vi "TOP BOTTOM Timestamp.vi"(4 "Format":enum16{"at TOP", "at BOTTOM", "none"}(ring), 5 "Plot Bounds":T2, 6 "Timestamp":dbl, 7 "pixel center":cluster{"horizontal":i16, "vertical":i16}, 8 "time format (%H:%M:%S)":string="%I:%M:%S %p", 9 "GraphBGK":u32(colorbox), 10 "font":T1, 11 "new picture in":picture) -> (3 "new picture out":picture)   [LabVIEW 2019]
uses:
  <vilib>/Utility/miscctls.llb/LVRectTypeDef.ctl
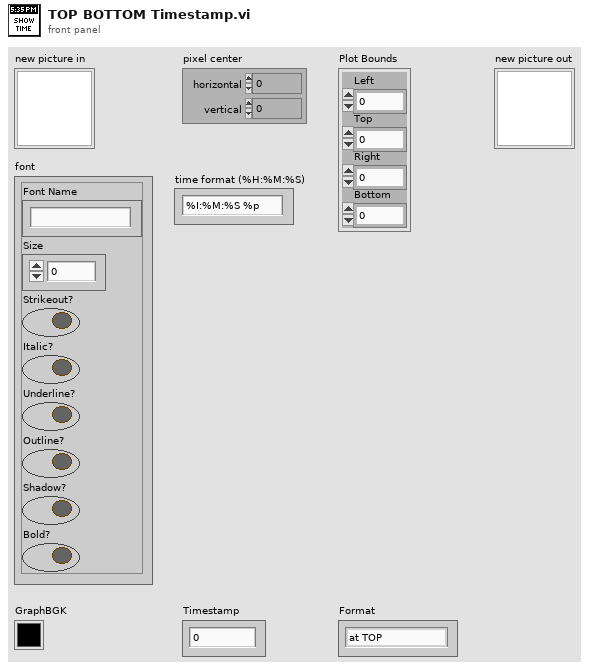
[diagram p1: front panel]
types:
  T1 = cluster{"Font Name":string, "Size":i16, "Strikeout?":bool, "Italic?":bool, "Underline?":bool, "Outline?":bool, "Shadow?":bool, "Bold?":bool}
  T2 = typedef "LVRectTypeDef.ctl" = cluster{"Left":i16, "Top":i16, "Right":i16, "Bottom":i16}
  T3 = enum16{"User-specified Font", "Application Font", "System Font", "Dialog Font"}
  T4 = cluster{"horizontal":enum16{"left", "center", "right"}, "vertical":enum16{"top", "center", "bottom"}}
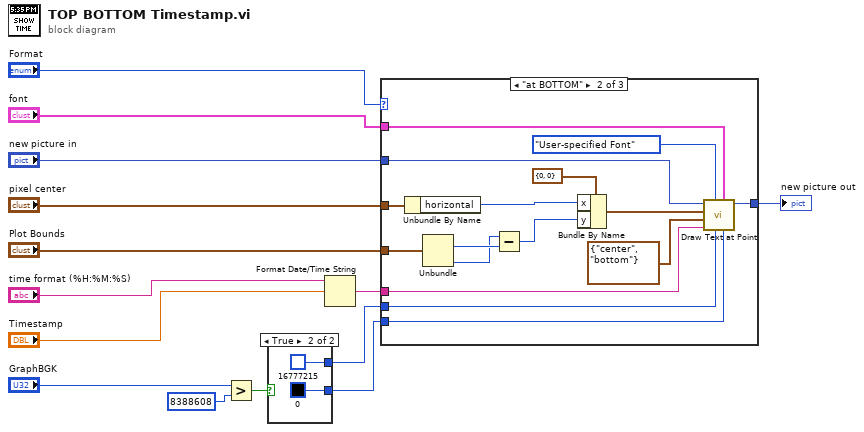
[diagram p0: block diagram]
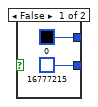
[diagram p2: hidden frame]
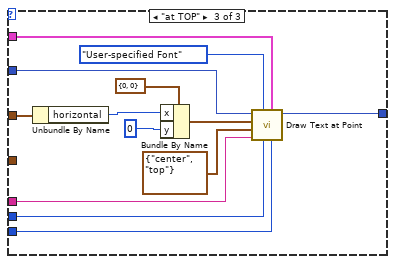
[diagram p4: hidden frame]
diagram:
  n1 = Greater?(x="GraphBGK", y=u32 8388608) -> (0:w9:bool)
  n2 = case shown="True" w9 {
    tunnel: [u32 0 u32 16777215] -> w6
    tunnel: [u32 16777215 u32 0] -> w5
    frame False {
    }
    frame True {
    }
  }
  n3 = Format Date/Time String(time format string (%c)="time format (%H:%M:%S)", seconds (now)="Timestamp") -> (date/time string=w1:string)  [unwired: 1 in]
  n4 = case shown="\"at BOTTOM\"" "Format" {
    tunnel: w1 -> [_ w20 w36]
    tunnel: "Plot Bounds" -> [_ w29 _]
    tunnel: "pixel center" -> [_ w28 w48]
    tunnel: [w19 w34 w46] -> w11
    tunnel: "new picture in" -> [w19 w33 w45]
    tunnel: w6 -> [_ w24 w40]
    tunnel: w5 -> [_ w23 w39]
    tunnel: "font" -> [_ w21 w38]
    frame "none" {
    }
    frame "at BOTTOM" {
      n5 = Unbundle By Name(w28) -> ("horizontal"=w31:i16)
      n6 = Unbundle(w29) -> ("Top"=w27:i16, "Bottom"=w26:i16)  [unwired: 2 out]
      n7 = Subtract(x=w26, y=w27) -> (x-y=w25:i16)
      n8 = Bundle By Name(cluster=cluster{"x":i16, "y":i16} {"x"=0, "y"=0} ("origin"), "x"=w31, "y"=w25) -> (w32:cluster{"x":i16, "y":i16})
      n9 = call <vilib>:"Draw Text at Point.vi"("BG color(transparent)"=w23, "[user-specified font]"=w21, "text color(black)"=w24, "desired font(Application)"=T3."User-specified Font", "text"=w20, "alignment(left, top)"=T4 {"horizontal"=enum."center", "vertical"=enum."bottom"}, "origin"=w32, "picture"=w33) -> ("new picture"=w34:picture)  [unwired: 2 in, 1 out]
    }
    frame "at TOP" {
      n10 = Unbundle By Name(w48) -> ("horizontal"=w43:i16)
      n11 = Bundle By Name(cluster=cluster{"x":i16, "y":i16} {"x"=0, "y"=0} ("origin"), "x"=w43, "y"=i16 0) -> (w44:cluster{"x":i16, "y":i16})
      n12 = call <vilib>:"Draw Text at Point.vi"("BG color(transparent)"=w39, "[user-specified font]"=w38, "text color(black)"=w40, "desired font(Application)"=T3."User-specified Font", "text"=w36, "alignment(left, top)"=T4 {"horizontal"=enum."center", "vertical"=enum."top"}, "origin"=w44, "picture"=w45) -> ("new picture"=w46:picture)  [unwired: 2 in, 1 out]
    }
  }
  "new picture out" <- w11
